vi "Update display current.vi"(8 "error in (no error)":errorcluster, 11 "StageSPIM in":refnum<class "StageSPIM.lvclass">) -> (0 "error out":errorcluster, 3 "StageSPIM out":refnum<class "StageSPIM.lvclass">)   [LabVIEW 2012, in "StageSPIM.lvclass"]
uses:
  StageSPIM.lvclass
  StageSPIM.lvclass/StageSPIM.ctl
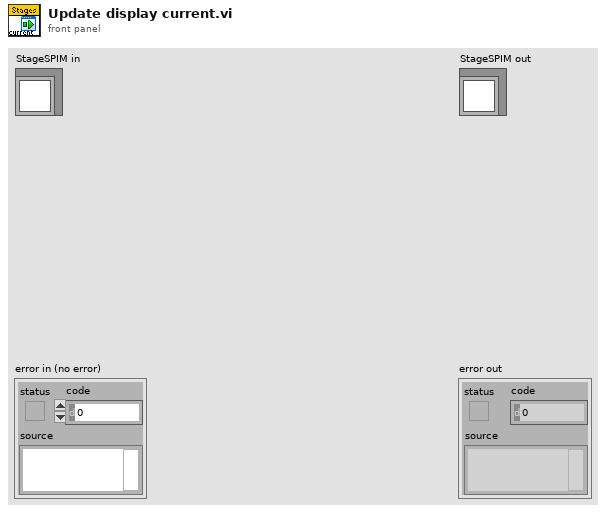
[diagram p1: front panel]
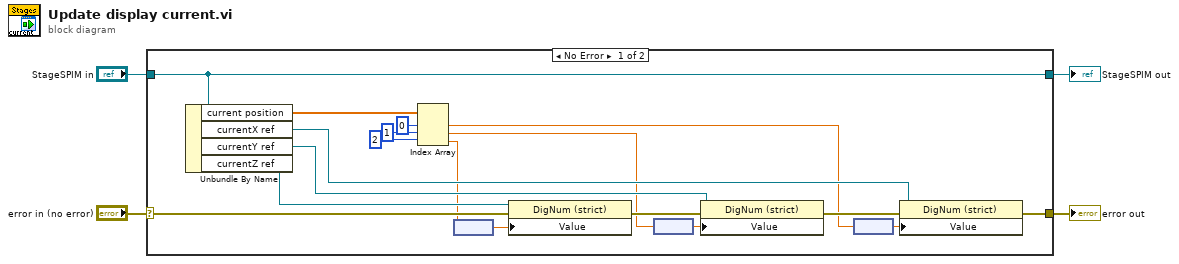
[diagram p0: block diagram]
diagram:
  n1 = case shown="No Error" "error in (no error)" {
    selector: "error in (no error)" -> [w17 w24]
    tunnel: [w8 w24] -> w3
    tunnel: [w22 w23] -> w1
    tunnel: "StageSPIM in" -> [w22 w23]
    frame No Error {
      n2 = Unbundle By Name(w22) -> ("current position"=w21:dbl[], "currentX ref"=w14:refnum<vi>, "currentY ref"=w15:refnum<vi>, "currentZ ref"=w16:refnum<vi>)
      n3 = Index Array(array=w21, index #1=0 ("index"), index #2=1 ("index"), index #3=2 ("index")) -> (element #1=w7:dbl, element #2=w6:dbl, element #3=w5:dbl)
      n4 = node(w5) -> (w11:dbl[unit])
      n5 = property class="DigNum (strict)"(reference=w16, error in=w17, "Value"=w11) -> (error out=w13:errorcluster)  [unwired: 1 out]
      n6 = node(w6) -> (w10:dbl[unit])
      n7 = property class="DigNum (strict)"(reference=w15, error in=w13, "Value"=w10) -> (error out=w12:errorcluster)  [unwired: 1 out]
      n8 = node(w7) -> (w9:dbl[unit])
      n9 = property class="DigNum (strict)"(reference=w14, error in=w12, "Value"=w9) -> (error out=w8:errorcluster)  [unwired: 1 out]
    }
    frame Error {
    }
  }
  "error out" <- w3
  "StageSPIM out" <- w1
